vi "XIPIN_XADC_Wizard_3_2.vi"   [LabVIEW 2017]
doc: "The XADC Wizard generates an HDL wrapper to configure a single 7 Series FPGA XADC primitive for user-specified channels and alarms.\n------------------------------------\n<b>Need License</b> : No\n<b>Interface</b> : AXI4 AXI4-Stream"
uses:
  <vilib>/rvi/XilinxIP/XIPIN_XNode/niFpgaXIPIN.xnode
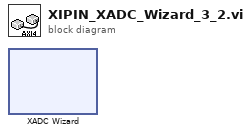
[diagram p0: block diagram]
diagram:
  n1 = xnode ("XADC Wizard")() -> ()
